vi "StringCallback.vi"(10 "String":string) -> ()   [LabVIEW 2013]
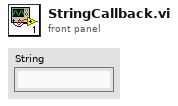
[diagram p1: front panel]
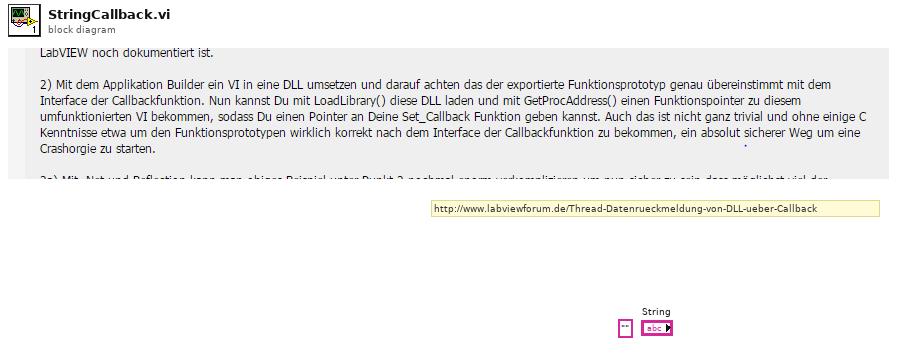
[diagram p0: block diagram]
diagram:
  (unwired) ""
  # "http://www.labviewforum.de/Thread-Datenrueckmeldung-von-DLL-ueber-Callback"
